vi "Instrument Delete.vi"(8 "error in (no error)":errorcluster, 10 "Instrument Record":T2, 11 "Connection Refnum":T1) -> (0 "error out":errorcluster, 3 "Connection Refnum":T1)   [LabVIEW 2011]
uses:
  Instrument Record.ctl
  SI.LIB/ODBC/SQL Controls/Connection Refnum.ctl
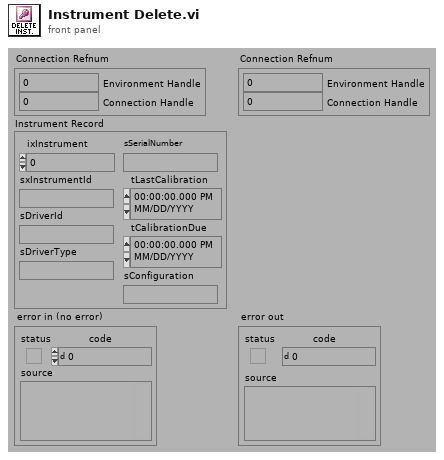
[diagram p1: front panel]
types:
  T1 = typedef "Connection Refnum.ctl" = cluster{"Environment Handle":i32, "Connection Handle":i32}
  T2 = typedef "Instrument Record.ctl" = cluster{"ixInstrument":i32, "sxInstrumentId":string, "sDriverId":string, "sDriverType":string, "sSerialNumber":string, "tLastCalibration":timestamp, "tCalibrationDue":timestamp, "sConfiguration":string}
  T3 = typedef "Statement Refnum.ctl" = cluster{"Statement Handle":i32, "Parameter Number":u16}
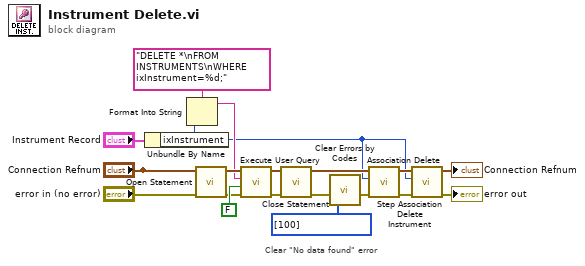
[diagram p0: block diagram]
diagram:
  # "Clear \"No data found\" error"
  n1 = Unbundle By Name("Instrument Record") -> ("ixInstrument"=w1:i32)
  n2 = Format Into String(format string="DELETE *\nFROM INSTRUMENTS\nWHERE ixInstrument=%d;" ("User Query"), w1) -> (resulting string=w11:string)  [unwired: 2 in, 1 out]
  n3 = call "Open Statement.vi"("error in (no error)"="error in (no error)", "Connection Refnum"="Connection Refnum") -> ("error out"=w13:errorcluster, "Statement Refnum"=w12:T3)  [unwired: 4 out]
  n4 = call "Execute User Query.vi"("error in (no error)"=w13, "Return Data? (f)"=FALSE, "User Query"=w11, "Statement Refnum"=w12) -> ("error out"=w15:errorcluster, "Statement Refnum"=w16:T3)  [unwired: 2 out]
  n5 = call "Close Statement.vi"("error in (no error)"=w15, "Statement Refnum"=w16) -> ("error out"=w9:errorcluster)  [unwired: 5 out]
  n6 = call "Clear Errors by Codes.vi"("Error Codes\nto Clear (Empty)"=i32[] [100] ("Error Codes\nto Clear (Empty)"), "error in (no error)"=w9) -> ("error out"=w8:errorcluster)  [unwired: 5 out]
  n7 = call "Association Delete.vi"("error in (no error)"=w8, "iInstrument (0)"=w1, "Connection Refnum"="Connection Refnum") -> ("error out"=w5:errorcluster, "Connection Refnum"=w2:T1)  [unwired: 1 in, 6 out]
  n8 = call "Step Association Delete Instrument.vi"("error in (no error)"=w5, "iInstrument (0)"=w1, "Connection Refnum"=w2) -> ("error out"=→"error out":errorcluster, "Connection Refnum"=→"Connection Refnum":T1)  [unwired: 7 in]
